vi "famtView.vi"   [LabVIEW 2015, in "FAMTViews.lvlib"]
uses:
  FAMTViews.lvlib
  CommandFactory/CommandFactory.lvclass
  UserEvents/UserEvents.lvclass
  UserEvents/UserEvents.lvclass/UserEvents.ctl
  Typedefs/CommandSelector.ctl
  Typedefs/StateSelector.ctl
  openLoopControlView.vi
  ILCOutputsView.vi
  Typedefs/FAMTTypedefs.lvlib
  Controller/Controller.lvclass
  ConfigurationThisComponent/ConfigurationThisComponent.lvclass
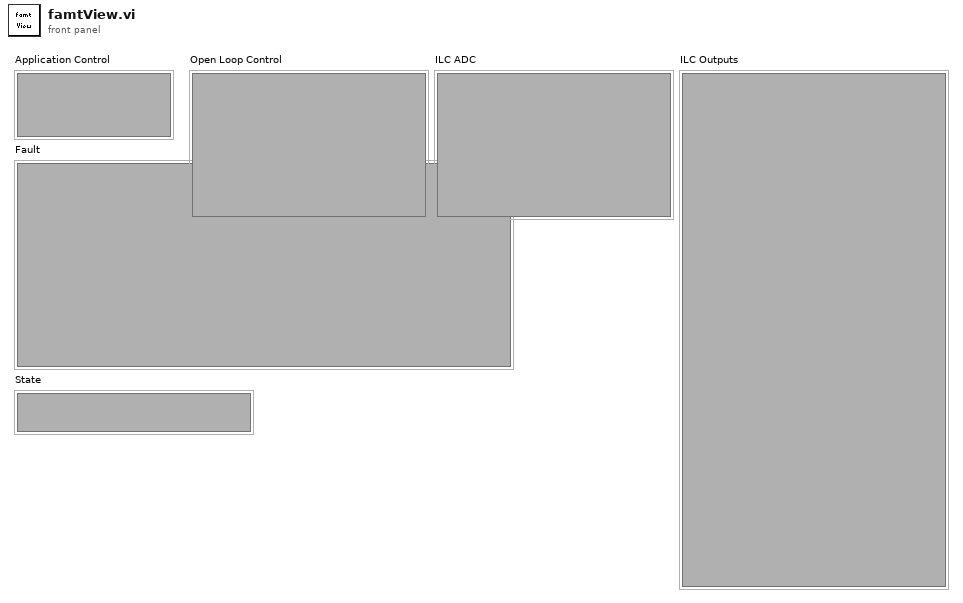
[diagram p1: front panel]
types:
  T1 = enum32{"invalid app kind", "Development System", "Run Time System", "Student Edition", "Embedded LabVIEW", "Evaluation", "Custom"}
  T2 = typedef "FAMTTypedefs.lvlib/PubDataEvents.ctl" = cluster{"State":refnum<user-event>, "ErrorCode":refnum<user-event>, "ADC Outputs":refnum<user-event>, "InputData":refnum<user-event>, "ControllerData":refnum<user-event>, "TestStatus":refnum<user-event>, "LogPath":refnum<user-event>, "ILC Outputs":refnum<user-event>}
  T3 = typedef "FAMTTypedefs.lvlib/SubDataEvents.ctl" = cluster{"Command":refnum<user-event>}
  T4 = cluster{"Event Registration Refnum":refnum<event-registration>, "Event Registration Refnum":refnum<event-registration>}
  T5 = typedef "FAMTTypedefs.lvlib/CommandSelector.ctl" = enum16{"Start", "Enable", "Disable", "Standby", "Shutdown", "Update"}
  T6 = typedef "FAMTTypedefs.lvlib/StateSelector.ctl" = enum16{"OfflineState", "FaultState", "StandbyState", "DisabledState", "EnabledState", "WaitForUserInputState", "PerformOpenLoopScanState"}
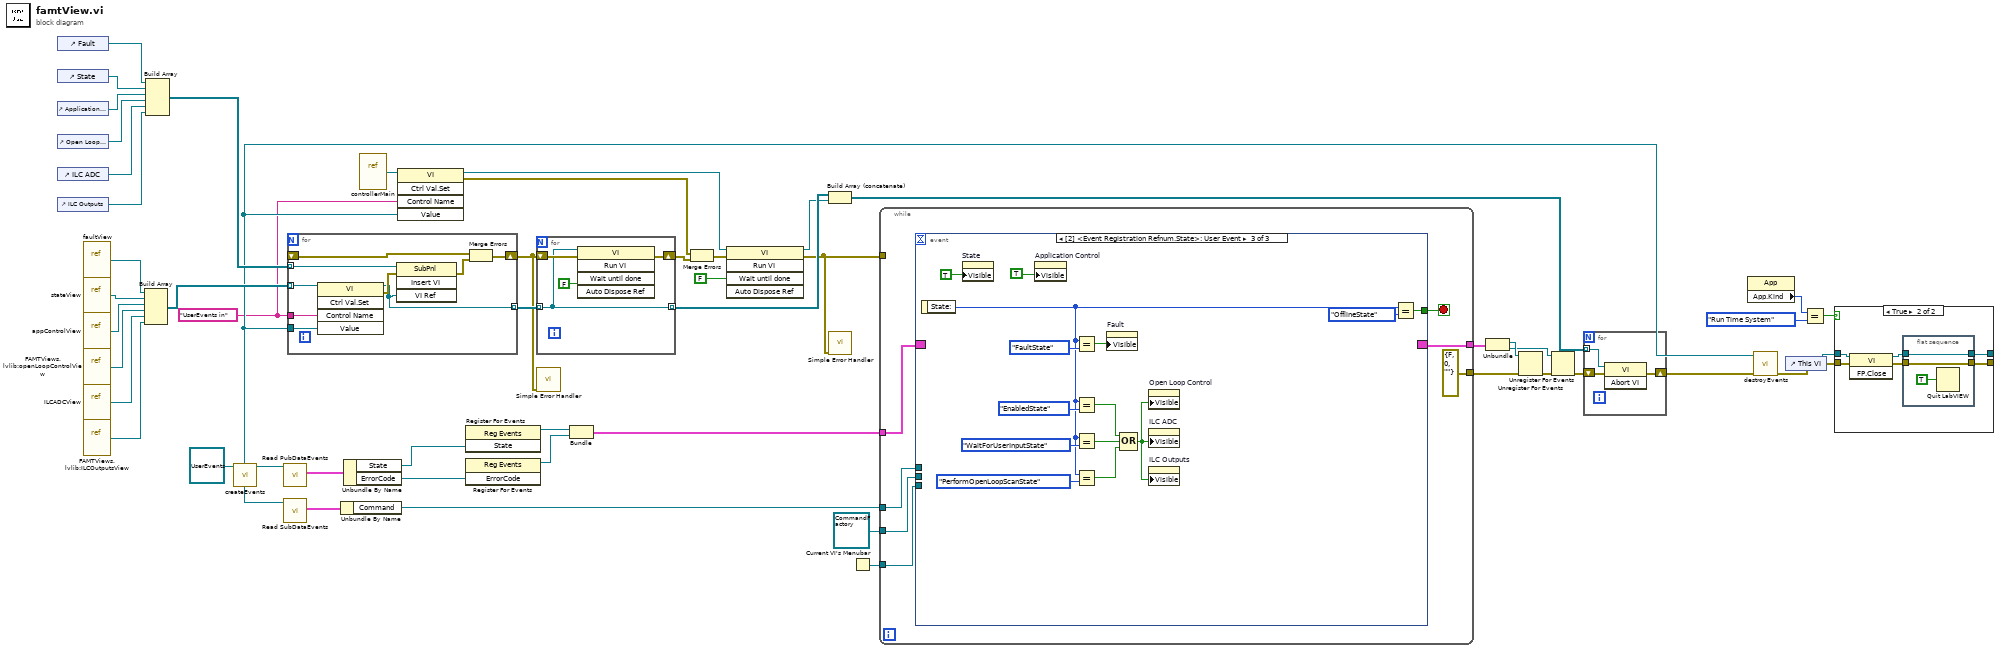
[diagram p0: block diagram]
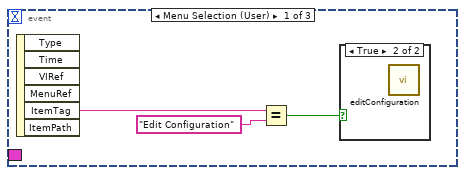
[diagram p3: hidden frame]
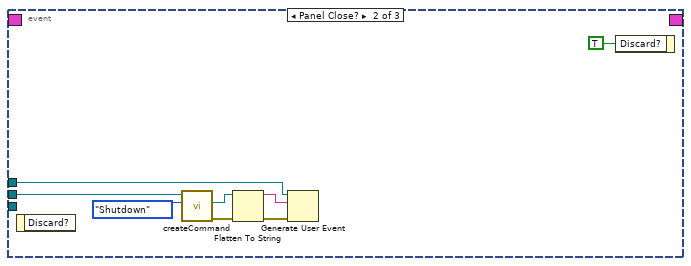
[diagram p5: hidden frame]
diagram:
  w15 = "UserEvents in" ("Control Name")
  n1 = control-ref of="Fault"() -> (w23:refnum<vi>)
  n2 = control-ref of="State"() -> (w24:refnum<vi>)
  n3 = control-ref of="Application Control"() -> (w25:refnum<vi>)
  n4 = control-ref of="Open Loop Control"() -> (w7:refnum<vi>)
  n5 = control-ref of="ILC ADC"() -> (w6:refnum<vi>)
  n6 = control-ref of="ILC Outputs"() -> (w1:refnum<vi>)
  n7 = vi-ref "faultView.vi"() -> (w22:refnum<vi>)
  n8 = vi-ref "stateView.vi"() -> (w21:refnum<vi>)
  n9 = vi-ref "appControlView.vi"() -> (w20:refnum<vi>)
  n10 = vi-ref "FAMTViews.lvlib:openLoopControlView.vi"() -> (w8:refnum<vi>)
  n11 = vi-ref "ILCADCView.vi"() -> (w3:refnum<vi>)
  n12 = vi-ref "FAMTViews.lvlib:ILCOutputsView.vi"() -> (w2:refnum<vi>)
  n13 = Build Array(w22, w21, w20, w8, w3, w2) -> (w18:refnum<vi>[])
  n14 = Build Array(w23, w24, w25, w7, w6, w1) -> (w19:refnum<vi>[])
  n15 = call "createEvents.vi"("UserEvents in"=refnum<class "UserEvents.lvclass"> refnum) -> ("UserEvents out"=w16:refnum<class "UserEvents.lvclass">)  [unwired: 9 in, 1 out]
  n16 = call "Read PubDataEvents.vi"("UserEvents in"=w16) -> ("PubDataEvents"=w46:T2)  [unwired: 9 in, 1 out]
  n17 = call "Read SubDataEvents.vi"("UserEvents in"=w16) -> ("SubDataEvents"=w44:T3)  [unwired: 9 in, 1 out]
  n18 = for {
    tunnel: w16 -> [w60]
    tunnel: w19 -> [w59] mode=indexing
    tunnel: w18 -> [w53] mode=indexing
    shift-right: [w58] -> w5
    shift-left: _ -> [w57]
    tunnel: [w52] -> w17 mode=indexing
    tunnel: w15 -> [w56]
    n19 = invoke class="VI" method="Ctrl Val.Set"(reference=w53, "Control Name"=w56, "Value"=w60) -> (reference out=w52:refnum<vi>, error out=w55:errorcluster)  [unwired: 2 in, 3 out]
    n20 = invoke on="Invoke Node" class="SubPnl" method="Insert VI"(reference=w59, error in=w55, "VI Ref"=w52) -> (error out=w54:errorcluster)  [unwired: 1 in, 3 out]
    n21 = Merge Errors(w57, w54) -> (w58:errorcluster)
  }
  n22 = Unbundle By Name(w44) -> ("Command"=w43:refnum<user-event>)
  n23 = Unbundle By Name(w46) -> ("State"=w42:refnum<user-event>, "ErrorCode"=w40:refnum<user-event>)
  n24 = vi-ref "controllerMain.vi"() -> (w37:refnum<vi>)
  n25 = invoke class="VI" method="Ctrl Val.Set"(reference=w37, "Control Name"=w15, "Value"=w16) -> (reference out=w36:refnum<vi>, error out=w12:errorcluster)  [unwired: 2 in, 3 out]
  n26 = register-events(w42) -> (reference out=w41:refnum<event-registration>)  [unwired: 2 in, 1 out]
  n27 = register-events(w40) -> (reference out=w39:refnum<event-registration>)  [unwired: 2 in, 1 out]
  n28 = for {
    shift-right: [w64] -> w14
    shift-left: w5 -> [w63]
    tunnel: w17 -> [w61] mode=indexing
    tunnel: [w61] -> w11 mode=indexing
    n29 = invoke class="VI" method="Run VI"(reference=w61, error in=w63, "Wait until done"=FALSE ("Wait Until Done")) -> (error out=w64:errorcluster)  [unwired: 2 in, 4 out]
  }
  n30 = call <vilib>:"Simple Error Handler.vi"("error in (no error)"=w5) -> ()  [unwired: 4 in, 5 out]
  n31 = Bundle("Event Registration Refnum"=w41, "Event Registration Refnum"=w39) -> (w34:T4)  [unwired: 1 in]
  n32 = Merge Errors(w12, w14) -> (w13:errorcluster)
  n33 = invoke class="VI" method="Run VI"(reference=w36, error in=w13, "Wait until done"=FALSE ("Wait Until Done")) -> (reference out=w10:refnum<vi>, error out=w4:errorcluster)  [unwired: 2 in, 3 out]
  n34 = Build Array (concatenate)(w11, w10) -> (w9:refnum<vi>[])
  n35 = call <vilib>:"Simple Error Handler.vi"("error in (no error)"=w4) -> ()  [unwired: 4 in, 5 out]
  n36 = Current VI's Menubar() -> (w47:refnum<k9>)
  n37 = while {
    tunnel: refnum<class "CommandFactory.lvclass"> refnum ("CommandFactory.lvclass") -> [w68]
    tunnel: [errorcluster {"status"=FALSE, "code"=0, "source"=""} ("error out")] -> w35
    tunnel: w47 -> [w66]
    tunnel: w34 -> [w70]
    tunnel: w43 -> [w67]
    tunnel: [w65] -> w33
    tunnel: w4 -> [_]
    stop <- w69 stop-if-true
    n38 = event shown="[2] <Event Registration Refnum.State>: User Event" {
      selector: w70 -> [_ _ _]
      dyn-events: [_ _ _] -> w65
      timeout: _ -> [_ _ _]
      tunnel: [_ _ w95] -> w69
      tunnel: w68 -> [_ w79 _]
      tunnel: w67 -> [_ w76 _]
      tunnel: w66 -> [_ _ _]
      event Menu Selection (User) {
        n39 = event-data() -> ("ItemTag"=w72:string)  [unwired: 1 in, 5 out]
        n40 = Equal?(x=w72, y="Edit Configuration") -> (x = y?=w74:bool)
        n41 = case shown="True" w74 {
          frame False {
          }
          frame True {
            n42 = call "editConfiguration.vi"() -> ()  [unwired: 10 in, 2 out]
          }
        }
      }
      event Panel Close? {
        n43 = event-data() -> ()  [unwired: 1 in, 1 out]
        n44 = call-dynamic "createCommand.vi"("Command"=CommandSelector."Shutdown", "CommandFactory in"=w79) -> ("error out"=w82:errorcluster, "command"=w81:refnum<class "Command.lvclass">)  [unwired: 7 in, 1 out]
        n45 = Flatten To String(anything=w81, error in (no error)=w82) -> (data string=w77:string, error out=w78:errorcluster)  [unwired: 2 in, 1 out]
        n46 = Generate User Event(user event=w76, event data cluster=w77, error in=w78) -> ()  [unwired: 1 in, 2 out]
        n47 = event-data("Discard?"=TRUE) -> ()  [unwired: 1 in, 1 out]
      }
      event User Event {
        n48 = event-data() -> ("State:"=w87:T6)  [unwired: 1 in]
        n49 = property on="State" class="SubPnl"("Visible"=TRUE) -> ()  [unwired: 2 in, 2 out]
        n50 = property on="Application Control" class="SubPnl"("Visible"=TRUE) -> ()  [unwired: 2 in, 2 out]
        n51 = Equal?(x=w87, y=StateSelector."FaultState") -> (x = y?=w91:bool)
        n52 = Equal?(x=w87, y=StateSelector."EnabledState") -> (x = y?=w86:bool)
        n53 = Equal?(x=w87, y=StateSelector."WaitForUserInputState") -> (x = y?=w85:bool)
        n54 = Equal?(x=w87, y=StateSelector."PerformOpenLoopScanState") -> (x = y?=w84:bool)
        n55 = property on="Fault" class="SubPnl"("Visible"=w91) -> ()  [unwired: 2 in, 2 out]
        n56 = Compound Arithmetic op=OR(w86, w85, w84) -> (w83:bool)
        n57 = property on="Open Loop Control" class="SubPnl"("Visible"=w83) -> ()  [unwired: 2 in, 2 out]
        n58 = property on="ILC ADC" class="SubPnl"("Visible"=w83) -> ()  [unwired: 2 in, 2 out]
        n59 = property on="ILC Outputs" class="SubPnl"("Visible"=w83) -> ()  [unwired: 2 in, 2 out]
        n60 = Equal?(x=w87, y=StateSelector."OfflineState") -> (x = y?=w95:bool)
      }
    }
  }
  n61 = Unbundle(w33) -> ("Event Registration Refnum"=w32:refnum<event-registration>, "Event Registration Refnum"=w30:refnum<event-registration>)
  n62 = Unregister For Events(event registration refnum=w32, error in=w35) -> (error out=w31:errorcluster)
  n63 = Unregister For Events(event registration refnum=w30, error in=w31) -> (error out=w29:errorcluster)
  n64 = for {
    tunnel: w9 -> [w97] mode=indexing
    shift-right: [w98] -> w28
    shift-left: w29 -> [w99]
    n65 = invoke class="VI" method="Abort VI"(reference=w97, error in=w99) -> (error out=w98:errorcluster)  [unwired: 1 in, 2 out]
  }
  n66 = property class="App"() -> ("App.Kind"=w51:T1)  [unwired: 2 in, 2 out]
  n67 = call "destroyEvents.vi"("error in (no error)"=w28, "UserEvents in"=w16) -> ("error out"=w26:errorcluster)  [unwired: 8 in, 1 out]
  n68 = control-ref of="This VI"() -> (w27:refnum<vi>)
  n69 = Equal?(x=w51, y=T1."Run Time System") -> (x = y?=w49:bool)
  n70 = case shown="True" w49 {
    tunnel: w27 -> [w101 w107]
    tunnel: w26 -> [w100 w106]
    tunnel: [w101 w104] -> _
    tunnel: [w100 w102] -> _
    frame False {
    }
    frame True {
      n71 = invoke class="VI" method="FP.Close"(reference=w107, error in=w106) -> (reference out=w103:refnum<vi>, error out=w105:errorcluster)  [unwired: 1 in, 1 out]
      n72 = flat-sequence {
        tunnel: w105 -> [w108]
        tunnel: [w109] -> w104
        tunnel: w103 -> [w109]
        tunnel: [w108] -> w102
        frame #0 {
          n73 = Quit LabVIEW(quit? (T)=TRUE) -> ()
        }
      }
    }
  }
